vi "General PID Simulator - 副本.vi"() -> ()   [LabVIEW 2022 SP3]
doc: "本范例演示如何仿真通用PID控制器。"
uses:
  <vilib>/addons/control/pid/pid.llb/PID (DBL).vi
  <vilib>/addons/control/pid/NI_PID_pid.lvlib
panel:
  out "操作变量":dbl(graph)
  in  "SP：":dbl(slide)=43.790849673202615 min=0.0 max=0.0 scale=0.0..100.0
  out "MV：":dbl(slide)=18.78965245852964 scale=-100.0..100.0
  out "PV：":dbl(slide)=60.754431603254424 scale=0.0..100.0
  in  "PID增益":T1={"比例增益(Kc)"=20.0, "积分时间（Ti，分）"=0.008, "微分时间（Td，分）"=0.001} {"微分时间（Td，分）" format="%.3f"; "积分时间（Ti，分）" format="%.3f"; "比例增益(Kc)" format="%.3f"}
  in  "停止":bool
  out "过程变量和设定值":cluster{"initial PV":dbl, "SP:":dbl}(graph)
  # "概述：本范例演示如何仿真简单PID循环控制器。\n操作步骤：\n1.运行VI，观察过程变量(PV)跟随设定值(SP)的值变化，同时控制器输出（也称作操作变量(MV)也发生变化，保持PV趋近SP值。\n2.稳定之后（PV逼近SP值），改变SP。移动显示控件上的蓝色箭头。MV变化，并再次使PV逼近SP。\n3.单击停止按钮停止VI。"
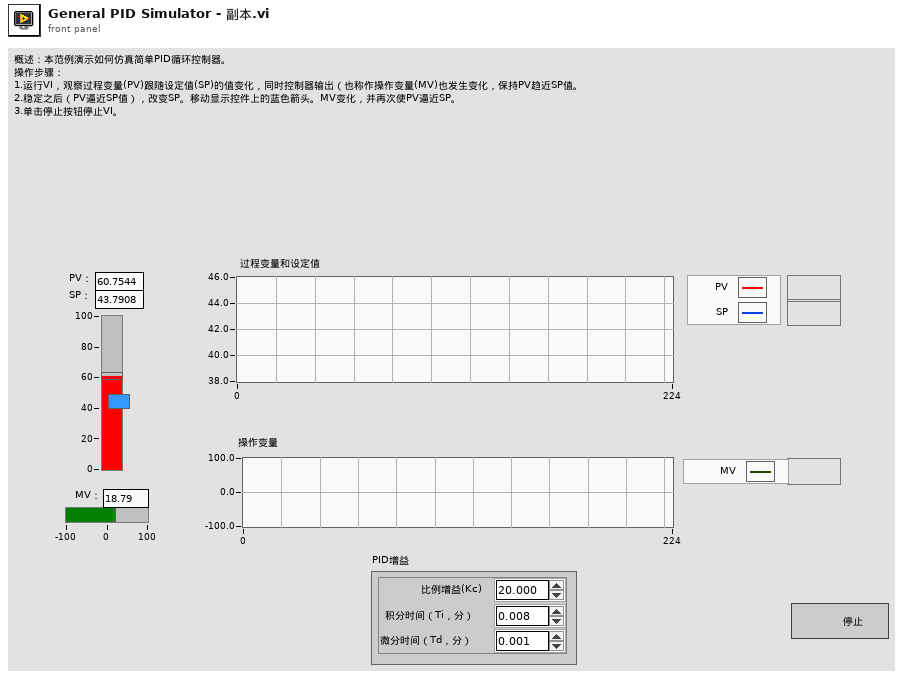
[diagram p1: front panel]
types:
  T1 = cluster{"比例增益(Kc)":dbl, "积分时间（Ti，分）":dbl, "微分时间（Td，分）":dbl}
  T2 = cluster{"static gain":dbl, "lag (min)":dbl, "dead cycles":dbl, "load %":dbl, "deadband":dbl, "noise level %":dbl, "initial PV":dbl, "initial PV 2":dbl}
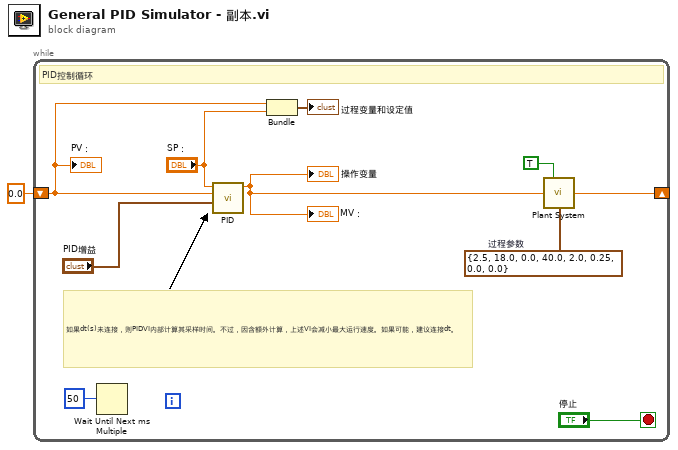
[diagram p0: block diagram]
diagram:
  n1 = while {
    shift-left: 0.0 ("Plant Output") -> [w8]
    shift-right: [w10] -> _
    stop <- "停止" stop-if-true
    w3 = T2 {"static gain"=2.5, "lag (min)"=18.0, "dead cycles"=0.0, "load %"=40.0, "deadband"=2.0, "noise level %"=0.25, "initial PV"=0.0, "initial PV 2"=0.0}  # 过程参数
    # "如果dt(s)未连接，则PIDVI内部计算其采样时间。不过，因含额外计算，上述VI会减小最大运行速度。如果可能，建议连接dt。"
    # "PID控制循环"
    n2 = Wait Until Next ms Multiple(millisecond multiple=u32 50 ("unsigned 32bit integer")) -> ()  [unwired: 1 out]
    n3 = call-poly <vilib>:"PID.vi"("PID gains"="PID增益", "process variable"=w8, "setpoint"="SP：") -> ("output"=w4:dbl)  [unwired: 7 in, 1 out]
    "MV：" <- w4
    "操作变量" <- w4
    n4 = Bundle("Plant Output"=w8, "SP："="SP：") -> (→"过程变量和设定值":cluster{"Plant Output":dbl, "SP：":dbl})  [unwired: 1 in]
    n5 = call "Plant System.vi"("积分器？"=TRUE ("Integrator ?"), "设备输入"=w4, "过程参数"=w3) -> ("设备输出"=w10:dbl)  [unwired: 12 in]
    "PV：" <- w8
  }
